vi "Read Config.ini Path.vi"(8 "error in (no error)":errorcluster, 11 "Configuration in":refnum<class "Configuration.lvclass">) -> (0 "error out":errorcluster, 2 "Config.ini Path":path, 3 "Configuration out":refnum<class "Configuration.lvclass">)   [LabVIEW 2018, in "Configuration.lvlib" / "Configuration.lvclass"]
doc: "This is returns the config.ini file path."
uses:
  Configuration.lvclass
  Configuration.lvclass/Configuration.ctl
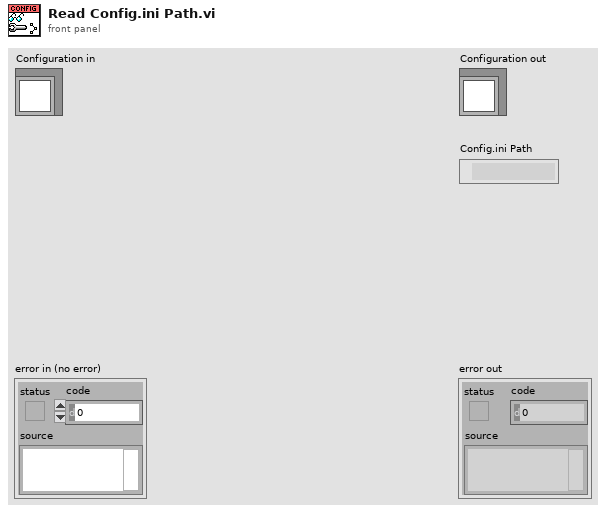
[diagram p1: front panel]
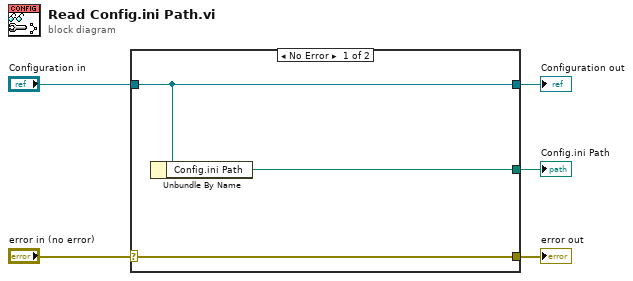
[diagram p0: block diagram]
diagram:
  n1 = case shown="No Error" "error in (no error)" {
    selector: "error in (no error)" -> [w8 w9]
    tunnel: [w8 w9] -> w4
    tunnel: [w7 w10] -> w2
    tunnel: "Configuration in" -> [w7 w10]
    tunnel: [w6 _] -> w1
    frame No Error {
      n2 = Unbundle By Name(w7) -> ("Config.ini Path"=w6:path)
    }
    frame Error {
    }
  }
  "error out" <- w4
  "Configuration out" <- w2
  "Config.ini Path" <- w1
